vi "LowerCuffButton.vi"(0 "error in":errorcluster, 2 "Side":T1, 3 "node":string) -> (1 "error out":errorcluster, 4 "Digital IO State":cluster{"state":i8, "is input only":bool})   [LabVIEW 2015]
uses:
  ROS/Code/SubVIs/BaxterSide.ctl
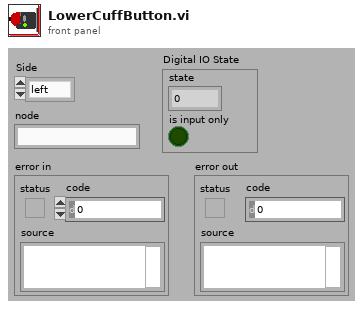
[diagram p1: front panel]
types:
  T1 = typedef "BaxterSide.ctl" = enum16{"left", "right"}
  T2 = enum16{"left_lower_cuff", "right_lower_cuff", "left_lower_button", "right_lower_button", "left_upper_button", "right_upper_button", "left_shoulder_button", "right_shoulder_button"}
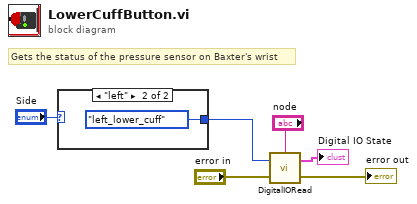
[diagram p0: block diagram]
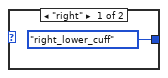
[diagram p2: hidden frame]
diagram:
  # "Gets the status of the pressure sensor on Baxter's wrist"
  n1 = case shown="\"left\"" "Side" {
    tunnel: [T2."right_lower_cuff" ("Component") T2."left_lower_cuff" ("Component")] -> w3
    frame "right" {
    }
    frame "left" {
    }
  }
  n2 = call "DigitalIORead.vi"("error in"="error in", "Component"=w3, "node"="node") -> ("error out"=→"error out":errorcluster, "Digital IO State"=→"Digital IO State":cluster{"state":i8, "is input only":bool})
